vi "CountToDistance (SubVI).vi"(11 "Counter Value":i32) -> (3 "Total Distance Travelled (m)":dbl)   [LabVIEW 2017]
panel:
  # "VI Name: CountToDistance (SubVI).vi\nAuthor: Steven Lee\n\nPlease see the corresponding block diagram for more detailed explanation."
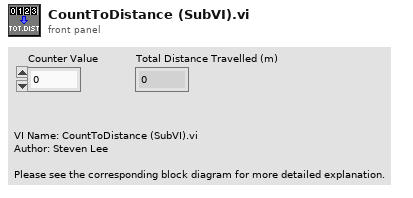
[diagram p1: front panel]
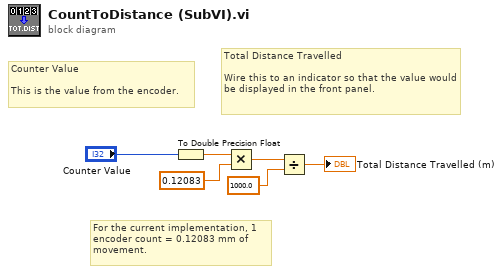
[diagram p0: block diagram]
diagram:
  # "Total Distance Travelled\n\nWire this to an indicator so that the value would be displayed in the front panel."
  # "For the current implementation, 1 encoder count = 0.12083 mm of movement."
  # "Counter Value\n\nThis is the value from the encoder."
  n1 = To Double Precision Float(number="Counter Value") -> (double precision float=w3:dbl)
  n2 = Multiply(x=w3, y=0.12083) -> (x*y=w4:dbl)
  n3 = Divide(x=w4, y=1000.0 ("x")) -> (x/y=→"Total Distance Travelled (m)":dbl)
